vi "Save Settings.vi"(8 "error in (no error)":errorcluster, 11 "Scanner in":refnum<class "Scanner.lvclass">) -> (0 "error out":errorcluster, 3 "Scanner out":refnum<class "Scanner.lvclass">)   [LabVIEW 2009, in "Scanner.lvclass"]
uses:
  Scanner.lvclass
  Scanner.lvclass/Scanner.ctl
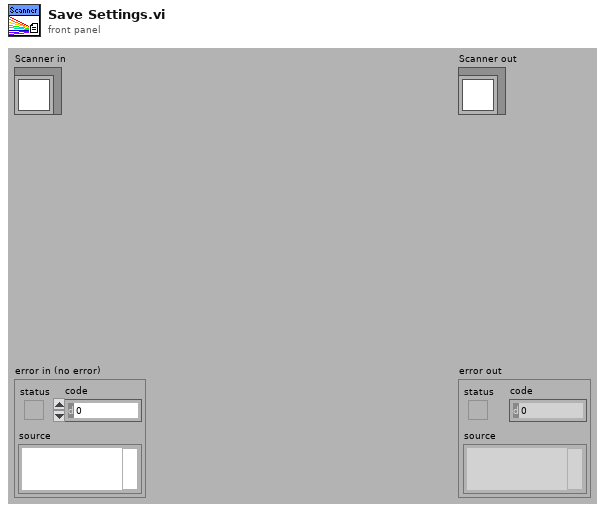
[diagram p1: front panel]
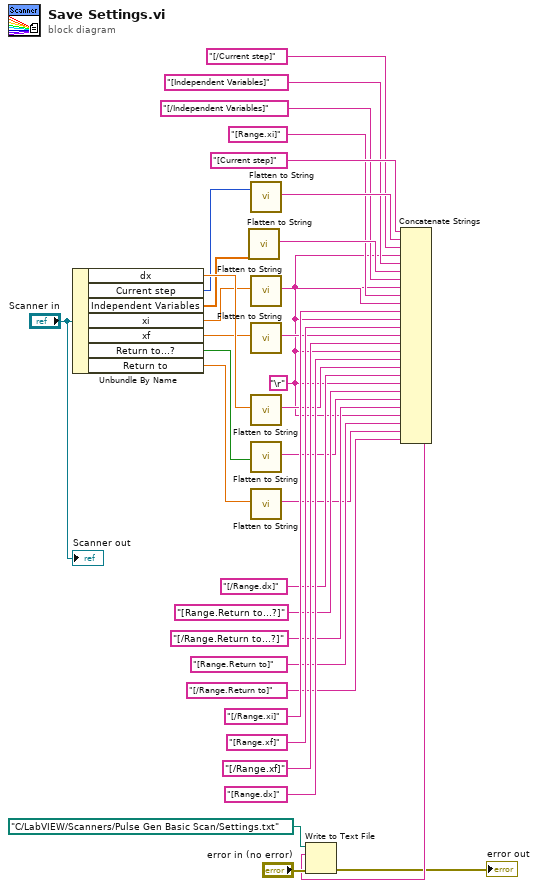
[diagram p0: block diagram]
diagram:
  w6 = "\r"
  n1 = Unbundle By Name("Scanner in") -> ("dx"=w31:dbl, "Current step"=w30:u32, "Independent Variables"=w29:dbl[], "xi"=w28:dbl, "xf"=w27:dbl, "Return to...?"=w26:bool, "Return to"=w25:dbl)
  n2 = call "Flatten to String.vi"("Array"=w29) -> ("Output String"=w20:string)  [unwired: 18 in]
  n3 = call "Flatten to String.vi"("I32"=w30) -> ("Output String"=w23:string)  [unwired: 18 in]
  n4 = call "Flatten to String.vi"("Float"=w28) -> ("Output String"=w17:string)  [unwired: 18 in]
  n5 = call "Flatten to String.vi"("Float"=w27) -> ("Output String"=w14:string)  [unwired: 18 in]
  n6 = call "Flatten to String.vi"("Float"=w31) -> ("Output String"=w11:string)  [unwired: 18 in]
  n7 = call "Flatten to String.vi"("Boolean"=w26) -> ("Output String"=w7:string)  [unwired: 18 in]
  n8 = call "Flatten to String.vi"("Float"=w25) -> ("Output String"=w3:string)  [unwired: 18 in]
  n9 = Concatenate Strings("[Current step]", w23, "[/Current step]", w6, "[Independent Variables]", w20, "[/Independent Variables]", w6, "[Range.xi]", w17, "[/Range.xi]", w6, "[Range.xf]", w14, "[/Range.xf]", w6, "[Range.dx]", w11, "[/Range.dx]", w6, "[Range.Return to...?]", w7, "[/Range.Return to...?]", w6, "[Range.Return to]", w3, "[/Range.Return to]") -> (w2:string)
  n10 = Write to Text File(file (use dialog)=path "C:/LabVIEW/Scanners/Pulse Gen Basic Scan/Settings.txt", text=w2, error in="error in (no error)") -> (error out=→"error out":errorcluster)  [unwired: 1 in, 2 out]
  "Scanner out" <- "Scanner in"
